vi "Example Pressure Control.vi"(1 "Stop":bool, 5 "error in (no error)":errorcluster, 7 "Pump Controller VISA resource name":refnum<visa-resource-name>, 9 "Pump Initial Flowrate, m^3/s":dbl, 11 "Pump Pressure, bar(G)":dbl format="%#_13g", 13 "Pump PID gains":T1={"proportional gain (Kc)"=1.0, "integral time (Ti, min)"=0.0, "derivative time (Td, min)"=0.0} {"derivative time (Td, min)" format="%.3f"; "integral time (Ti, min)" format="%.3f"; "proportional gain (Kc)" format="%.3f"}) -> (19 "error out":errorcluster)   [LabVIEW 2017]
uses:
  <vilib>/addons/control/pid/pid.llb/PID (DBL).vi
  <instrlib>/Roboteq Controller KBL1xxx/Roboteq Controller KBL1xxx.lvlib
  Pump Controller.lvlib
  <vilib>/addons/control/pid/NI_PID_pid.lvlib
panel:
  out "Pump Flowrate":dbl(graph)
  out "PID output":dbl(graph)
  out "Measured Pressure":dbl(graph)
  # "TODO: Read real pressure value in RUN state"
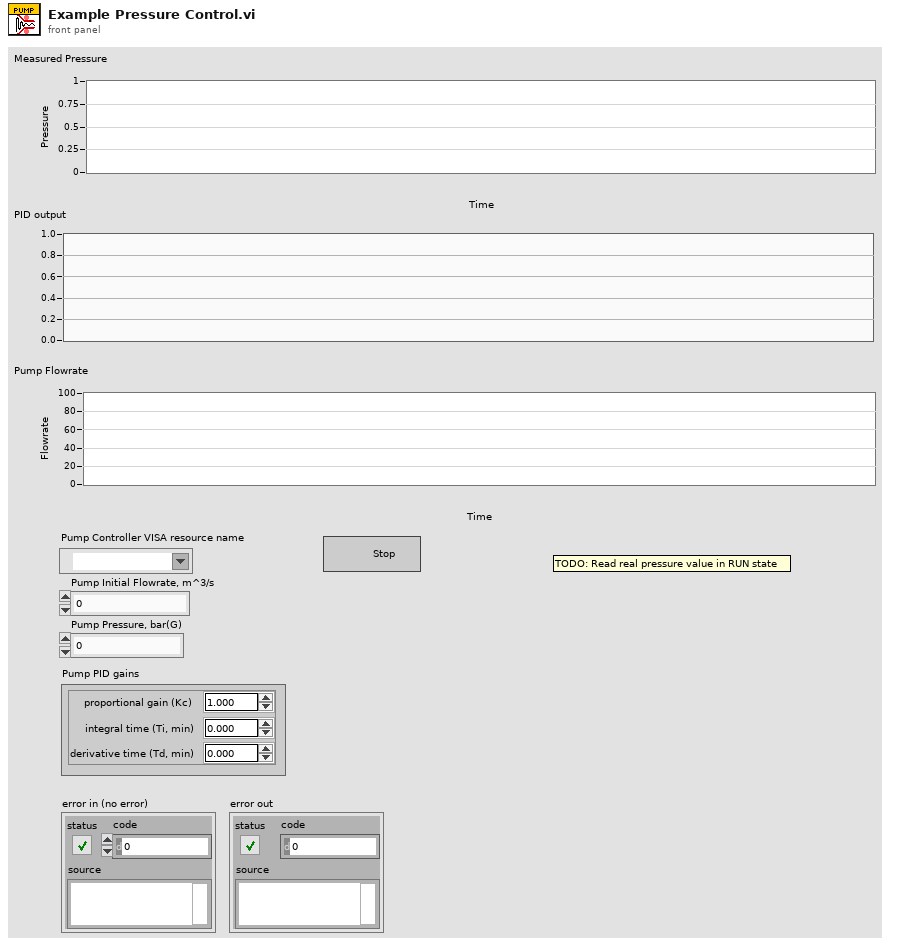
[diagram p1: front panel]
types:
  T1 = cluster{"proportional gain (Kc)":dbl, "integral time (Ti, min)":dbl, "derivative time (Td, min)":dbl}
  T2 = typedef "Roboteq Controller KBL1xxx.lvlib/Controller.ctl" = cluster{"VISA resource name out":refnum<visa-resource-name>, "MXRPM":u16}
  T3 = typedef "Pump Controller.lvlib/Pump.ctl" = cluster{"Controller":T2}
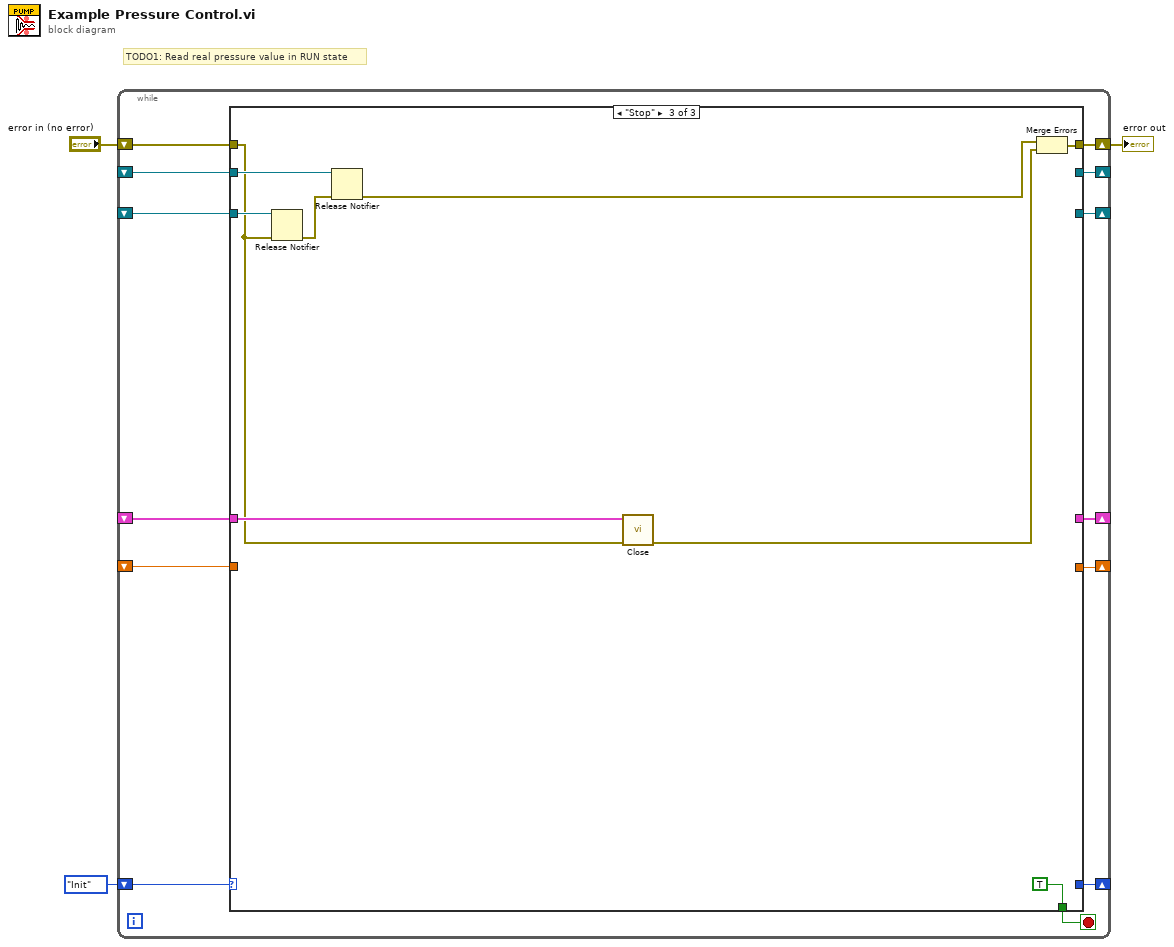
[diagram p0: block diagram]
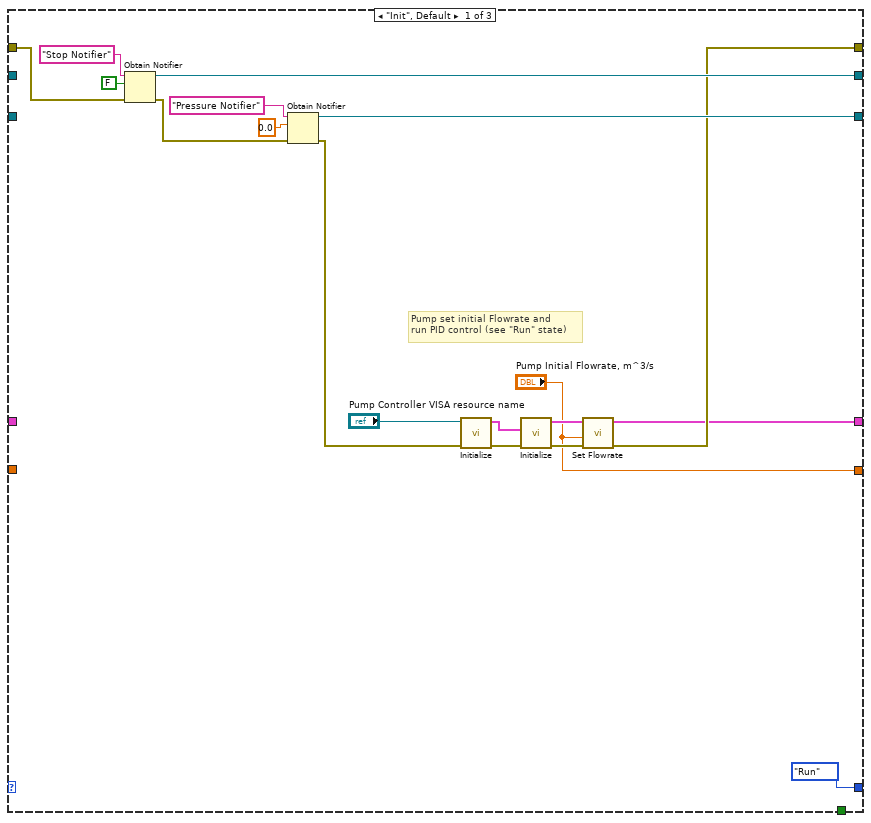
[diagram p2: hidden frame]
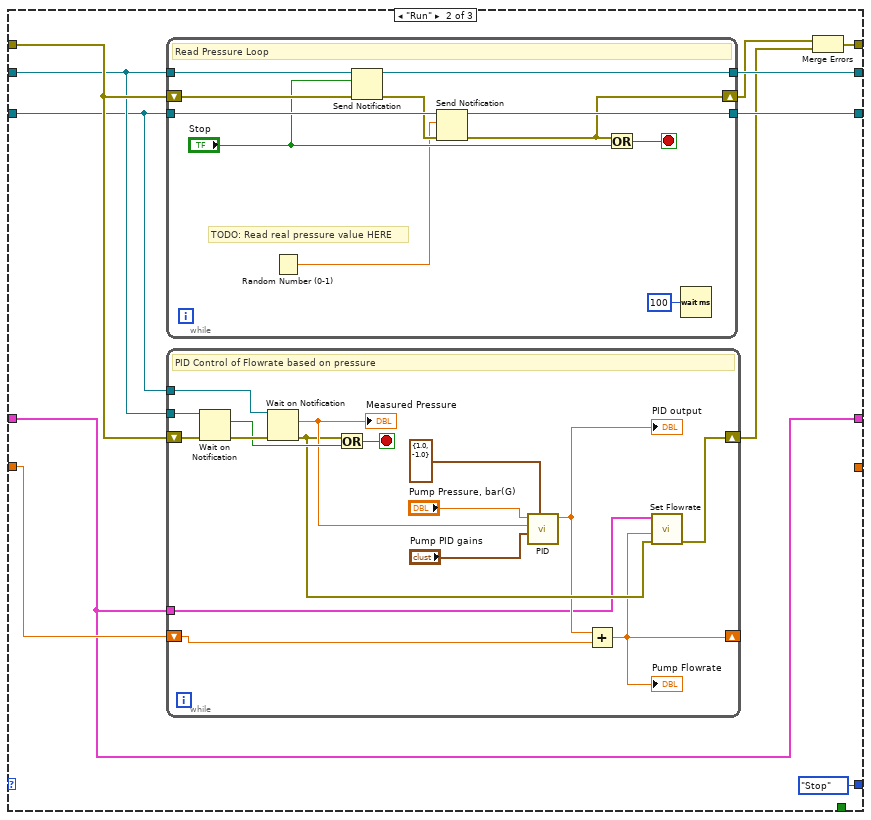
[diagram p3: hidden frame]
diagram:
  # "TODO1: Read real pressure value in RUN state"
  n1 = while {
    shift-right: [w15] -> _
    shift-left: enum16{"Init", "Run", "Stop"}."Init" ("State") -> [w16]
    shift-right: [w13] -> _
    shift-left: _ -> [w10]
    shift-right: [w12] -> _
    shift-left: _ -> [w9]
    shift-right: [w8] -> w1
    shift-left: "error in (no error)" -> [w11]
    shift-right: [w7] -> _
    shift-left: _ -> [w6]
    shift-right: [w5] -> _
    shift-left: _ -> [w4]
    stop <- w14 stop-if-true
    n2 = case shown="\"Stop\"" w16 {
      tunnel: [enum16{"Init", "Run", "Stop"}."Run" ("State") enum16{"Init", "Run", "Stop"}."Stop" ("State") _] -> w15
      tunnel: [_ _ TRUE] -> w14
      tunnel: [w28 w43 _] -> w13
      tunnel: [w27 w42 _] -> w12
      tunnel: w11 -> [w25 w44 w74]
      tunnel: w10 -> [_ w41 w78]
      tunnel: w9 -> [_ w40 w79]
      tunnel: [w20 w39 w76] -> w8
      tunnel: [w19 w35 _] -> w7
      tunnel: w6 -> [_ w35 w77]
      tunnel: ["Pump Initial Flowrate, m^3/s" _ _] -> w5
      tunnel: w4 -> [_ w36 _]
      frame "Init", Default {
        # "Pump set initial Flowrate and \nrun PID control (see \"Run\" state)"
        n3 = Obtain Notifier(name (unnamed)="Stop Notifier", notification data type=FALSE, error in (no error)=w25) -> (notifier out=w28:refnum<notifier>, error out=w33:errorcluster)  [unwired: 1 in, 1 out]
        n4 = Obtain Notifier(name (unnamed)="Pressure Notifier", notification data type=0.0, error in (no error)=w33) -> (notifier out=w27:refnum<notifier>, error out=w17:errorcluster)  [unwired: 1 in, 1 out]
        n5 = call <instrlib>:"Initialize.vi"("error in (no error)"=w17, "VISA resource name"="Pump Controller VISA resource name") -> ("error out"=w24:errorcluster, "Controller"=w23:T2)  [unwired: 8 in]
        n6 = call <instrlib>:"Initialize.vi"("error in (no error)"=w24, "Controller"=w23) -> ("error out"=w22:errorcluster, "Pump"=w21:T3)  [unwired: 8 in]
        n7 = call "Set Flowrate.vi"("error in (no error)"=w22, "Flowrate, m^3/s"="Pump Initial Flowrate, m^3/s", "Pump in"=w21) -> ("error out"=w20:errorcluster, "Pump out"=w19:T3)  [unwired: 7 in]
      }
      frame "Run" {
        n8 = while {
          tunnel: w41 -> [w71]
          tunnel: [w69] -> w43
          tunnel: w40 -> [w68]
          tunnel: [w66] -> w42
          shift-right: [w65] -> w38
          shift-left: w44 -> [w70]
          stop <- w63 stop-if-true
          # "TODO: Read real pressure value HERE"
          # "Read Pressure Loop"
          n9 = Random Number (0-1)() -> (number: 0 to 1=w62:dbl)
          n10 = Send Notification(notification="Stop", notifier=w71, error in (no error)=w70) -> (notifier out=w69:refnum<notifier>, error out=w67:errorcluster)
          n11 = Send Notification(notification=w62, notifier=w68, error in (no error)=w67) -> (notifier out=w66:refnum<notifier>, error out=w65:errorcluster)
          n12 = Or(x=w65, y="Stop") -> (x .or. y?=w63:bool)
          n13 = Wait (ms)(milliseconds to wait=u32 100) -> ()  [unwired: 1 out]
        }
        n14 = while {
          tunnel: w41 -> [w60]
          tunnel: w40 -> [w58]
          shift-right: [w51] -> w37
          shift-left: w44 -> [w61]
          shift-right: [w47] -> _
          shift-left: w36 -> [w48]
          tunnel: w35 -> [w46]
          stop <- w56 stop-if-true
          # "PID Control of Flowrate based on pressure"
          n15 = Wait on Notification(notifier=w60, error in (no error)=w61) -> (notification=w57:bool, error out=w59:errorcluster)  [unwired: 2 in, 2 out]
          n16 = Wait on Notification(notifier=w58, error in (no error)=w59) -> (notification=w54:dbl, error out=w52:errorcluster)  [unwired: 2 in, 2 out]
          "Measured Pressure" <- w54
          n17 = Or(x=w52, y=w57) -> (x .or. y?=w56:bool)
          n18 = call-poly <vilib>:"PID.vi"("output range"=cluster{"output high":dbl, "output low":dbl} {"output high"=1.0, "output low"=-1.0}, "PID gains"="Pump PID gains", "process variable"=w54, "setpoint"="Pump Pressure, bar(G)") -> ("output"=w49:dbl)  [unwired: 6 in, 1 out]
          "PID output" <- w49
          n19 = Add(x=w49, y=w48) -> (x+y=w47:dbl)
          "Pump Flowrate" <- w47
          n20 = call "Set Flowrate.vi"("error in (no error)"=w52, "Flowrate, m^3/s"=w47, "Pump in"=w46) -> ("error out"=w51:errorcluster)  [unwired: 7 in, 1 out]
        }
        n21 = Merge Errors(w38, w37) -> (w39:errorcluster)
      }
      frame "Stop" {
        n22 = Release Notifier(notifier=w79, error in (no error)=w74) -> (error out=w80:errorcluster)  [unwired: 1 in, 2 out]
        n23 = Release Notifier(notifier=w78, error in (no error)=w80) -> (error out=w75:errorcluster)  [unwired: 1 in, 2 out]
        n24 = call "Close.vi"("error in (no error)"=w74, "Pump in"=w77) -> ("error out"=w73:errorcluster)  [unwired: 9 in]
        n25 = Merge Errors(w75, w73) -> (w76:errorcluster)
      }
    }
  }
  "error out" <- w1
